vi "Initialization_Of_FGV.vi"(11 "expIndex":i32) -> ()   [LabVIEW 2020]
uses:
  Configuration/Global_Configurations.vi
panel:
  out "expIndex":i32
  out "expIndex":i32
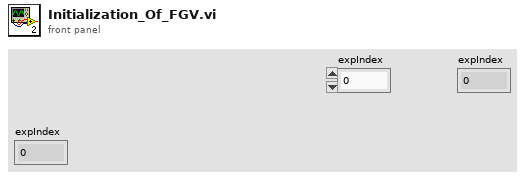
[diagram p1: front panel]
types:
  T1 = cluster{"Path":path, "Name":string, "Authors":string, "Keywords":string, "Description":string, "Cameras":cluster{"Base URL":string, "Path":string, "Name":string}[], "Sampling":cluster{"Sampled Variable":string, "Delta":dbl}[], "Sampling Freq":u32}[]
  T2 = cluster{"Path":path, "Name":string, "Authors":string, "Keywords":string, "Description":string, "Cameras":cluster{"Base URL":string, "Path":string, "Name":string}[], "Sampling":cluster{"Sampled Variable":string, "Delta":dbl}[], "Sampling Freq":u32}
  T3 = cluster{"Sampled Variable":string, "Delta":dbl}[]
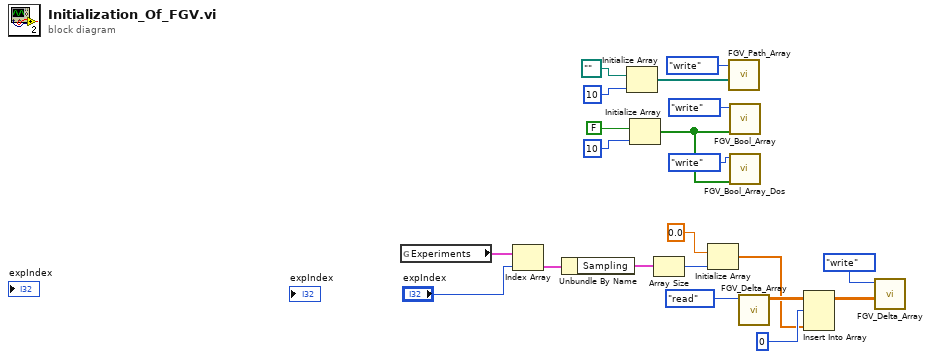
[diagram p0: block diagram]
diagram:
  n1 = global read "Global_Configurations.vi" "Experiments"() -> (w12:T1)
  n2 = Index Array(array=w12, index="expIndex") -> (element=w11:T2)
  n3 = Unbundle By Name(w11) -> ("Sampling"=w10:T3)
  n4 = Initialize Array(path "", 10) -> (w21:path[])
  n5 = Initialize Array(FALSE, 10) -> (w17:bool[])
  n6 = Array Size(array=w10) -> (size(s)=w8:i32)
  n7 = Initialize Array(0.0, w8) -> (w2:dbl[])
  n8 = call "FGV_Path_Array.vi"("path in"=w21, "Enum"=enum16{"read", "write"}."write" ("operation (0:open)")) -> ()  [unwired: 9 in, 1 out]
  n9 = call "FGV_Bool_Array.vi"("Array In"=w17, "Enum"=enum16{"read", "write"}."write") -> ()  [unwired: 9 in, 1 out]
  n10 = call "FGV_Bool_Array_Dos.vi"("Array In"=w17, "Enum"=enum16{"read", "write"}."write" ("operation (0:open)")) -> ()  [unwired: 9 in, 1 out]
  n11 = call "FGV_Delta_Array.vi"("Enum"=enum16{"read", "write"}."read" ("operation (0:open)")) -> ("array out"=w7:dbl[][])  [unwired: 10 in]
  n12 = Insert Into Array(array=w7, index (row)=0, new element=w2) -> (w6:dbl[][])  [unwired: 1 in]
  n13 = call "FGV_Delta_Array.vi"("array in"=w6, "Enum"=enum16{"read", "write"}."write" ("operation (0:open)")) -> ()  [unwired: 9 in, 1 out]
